vi "DAQmx.Enumerate Devices.vi"(8 "error in (no error)":errorcluster) -> (0 "error out":errorcluster, 3 "Devices":T1[](array[typedef]))   [LabVIEW 2019, in "DAQmx.lvclass"]
uses:
  DAQmx.lvclass
  typedefs/DeviceInfo--Cluster.ctl
  <vilib>/numeric/Random Number (Range) U64.vi
  <vilib>/numeric/sub_Random U32.vi
  <resource>/objmgr/daqmx.rc
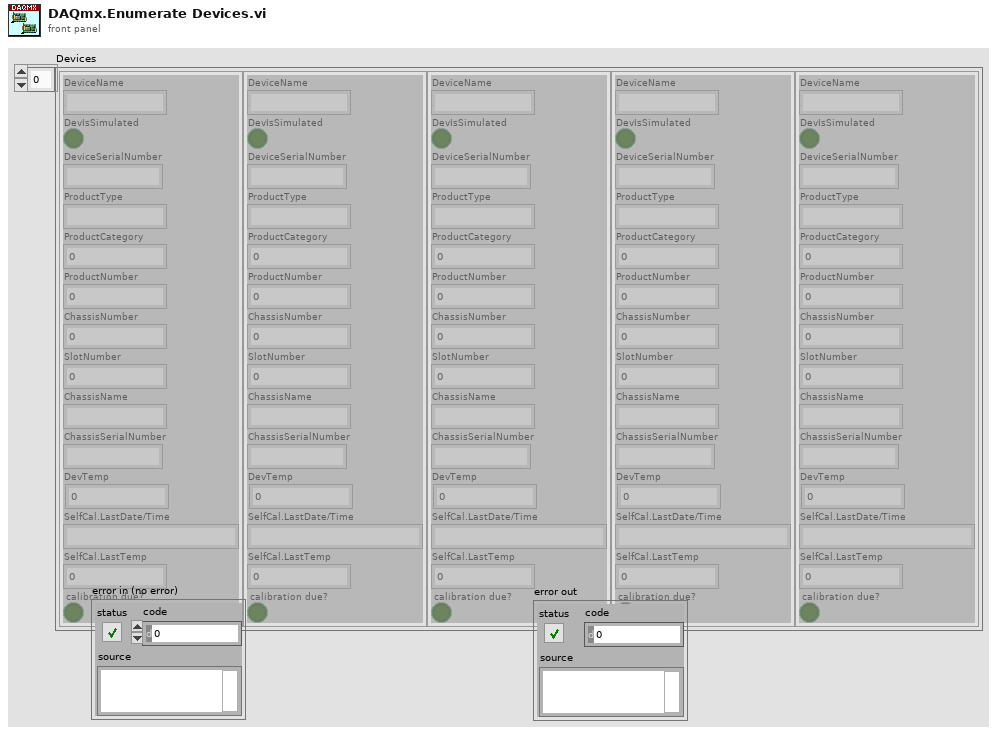
[diagram p1: front panel]
types:
  T1 = typedef "DAQmx.lvclass/DeviceInfo--Cluster.ctl" = cluster{"DeviceName":string, "DevIsSimulated":bool, "DeviceSerialNumber":string, "ProductType":string, "ProductCategory":i32, "ProductNumber":u32, "ChassisNumber":u32, "SlotNumber":u32, "ChassisName":string, "ChassisSerialNumber":string, "DevTemp":dbl, "SelfCal.LastDate/Time":string, "SelfCal.LastTemp":dbl, "calibration due?":bool}
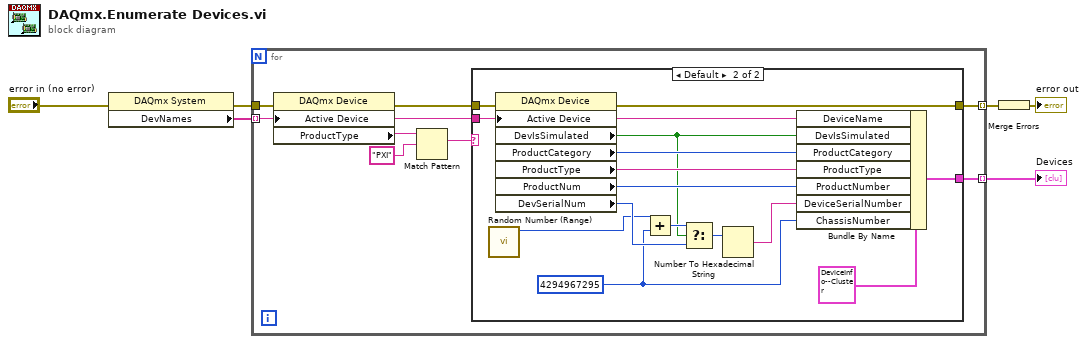
[diagram p0: block diagram]
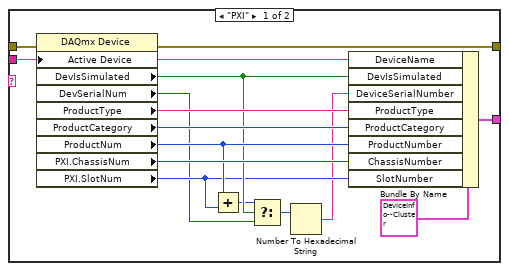
[diagram p2: hidden frame]
diagram:
  n1 = property class="DAQmx System"(error in="error in (no error)") -> (error out=w2:errorcluster, "DevNames"=w3:tag[])  [unwired: 1 in, 1 out]
  n2 = for {
    tunnel: w3 -> [w11] mode=indexing
    tunnel: w2 -> [w14]
    tunnel: [w7] -> w4 mode=indexing
    tunnel: [w8] -> w6 mode=indexing
    n3 = property class="DAQmx Device"(error in=w14, "Active Device"=w11) -> (error out=w10:errorcluster, "ProductType"=w13:string)  [unwired: 1 in, 1 out]
    n4 = Match Pattern(string=w13, regular expression="PXI") -> (match substring=w9:string)  [unwired: 1 in, 3 out]
    n5 = case shown="Default" w9 {
      tunnel: w10 -> [w29 w43]
      tunnel: [w28 w44] -> w7
      tunnel: w11 -> [w27 w41]
      tunnel: [w26 w40] -> w8
      frame "PXI" {
        n6 = property class="DAQmx Device"(error in=w29, "Active Device"=w27) -> (error out=w28:errorcluster, "DevIsSimulated"=w20:bool, "DevSerialNum"=w17:u32, "ProductType"=w22:string, "ProductCategory"=w23:i32, "ProductNum"=w21:u32, "PXI.ChassisNum"=w24:u32, "PXI.SlotNum"=w18:u32)  [unwired: 1 in, 1 out]
        n7 = Add(x=w21, y=w18) -> (x+y=w19:u32)
        n8 = Select(t=w19, s=w20, f=w17) -> (s? t:f=w16:u32)
        n9 = Number To Hexadecimal String(2:w16) -> (0:w15:string)  [unwired: 1 in]
        n10 = Bundle By Name(cluster=T1 {"DeviceName"="", "DevIsSimulated"=FALSE, "DeviceSerialNumber"="", "ProductType"="", "ProductCategory"=0, "ProductNumber"=0, "ChassisNumber"=0, "SlotNumber"=0, "ChassisName"="", "ChassisSerialNumber"="", "DevTemp"=0.0, "SelfCal.LastDate/Time"="", "SelfCal.LastTemp"=0.0, "calibration due?"=FALSE} ("Device"), "DeviceName"=w27, "DevIsSimulated"=w20, "DeviceSerialNumber"=w15, "ProductType"=w22, "ProductCategory"=w23, "ProductNumber"=w21, "ChassisNumber"=w24, "SlotNumber"=w18) -> (w26:T1)
      }
      frame Default {
        w32 = u32 4294967295 ("PXI.ChassisNum")
        n11 = call-poly <vilib>:"Random Number (Range).vi"() -> ("number"=w31:u64)  [unwired: 11 in]
        n12 = property class="DAQmx Device"(error in=w43, "Active Device"=w41) -> (error out=w44:errorcluster, "DevIsSimulated"=w34:bool, "ProductCategory"=w38:i32, "ProductType"=w39:string, "ProductNum"=w37:u32, "DevSerialNum"=w33:u32)  [unwired: 1 in, 1 out]
        n13 = Add(x=w31, y=w32) -> (x+y=w36:u64)
        n14 = Select(t=w36, s=w34, f=w33) -> (s? t:f=w35:u64)
        n15 = Number To Hexadecimal String(2:w35) -> (0:w30:string)  [unwired: 1 in]
        n16 = Bundle By Name(cluster=T1 {"DeviceName"="", "DevIsSimulated"=FALSE, "DeviceSerialNumber"="", "ProductType"="", "ProductCategory"=0, "ProductNumber"=0, "ChassisNumber"=0, "SlotNumber"=0, "ChassisName"="", "ChassisSerialNumber"="", "DevTemp"=0.0, "SelfCal.LastDate/Time"="", "SelfCal.LastTemp"=0.0, "calibration due?"=FALSE} ("Device"), "DeviceName"=w41, "DevIsSimulated"=w34, "ProductCategory"=w38, "ProductType"=w39, "ProductNumber"=w37, "DeviceSerialNumber"=w30, "ChassisNumber"=w32) -> (w40:T1)
      }
    }
  }
  "Devices" <- w6
  n17 = Merge Errors(w4) -> (→"error out":errorcluster)
